vi "LINC Compile Sim Ops.vi"(1 "item formats":T2[](array[typedef])) -> (0 "sim ops":T1[](array[typedef]) {"mask" format="%02x"})   [LabVIEW 2018, in "STEPkgDriver_LINC.lvlib"]
uses:
  STEPkgDriver_LINC.lvlib
  LINC Sim Ops.ctl
  LINC Format Prototype.ctl
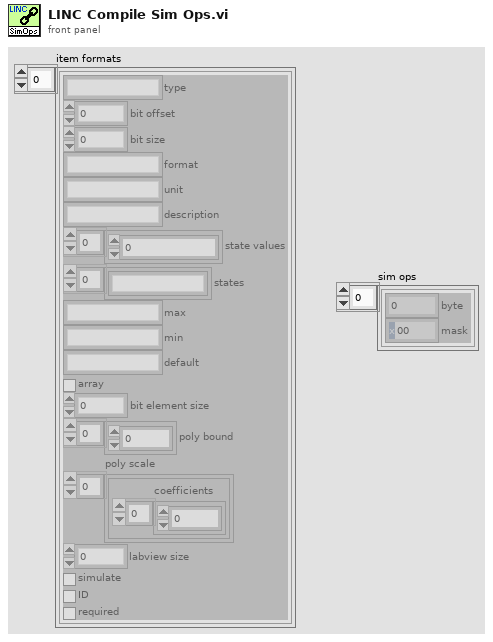
[diagram p1: front panel]
types:
  T1 = typedef "STEPkgDriver_LINC.lvlib/LINC Sim Ops.ctl" = cluster{"byte":i32, "mask":u8}
  T2 = typedef "STEPkgDriver_LINC.lvlib/LINC Format Prototype.ctl" = cluster{"type":string, "bit offset":i32, "bit size":i32, "format":string, "unit":string, "description":string, "state values":i64[], "states":string[], "max":string, "min":string, "default":string, "array":bool, "bit element size":i32, "poly bound":dbl[], "poly scale":cluster{"coefficients":dbl[]}[], "labview size":i32, "simulate":bool, "ID":bool, "required":bool}
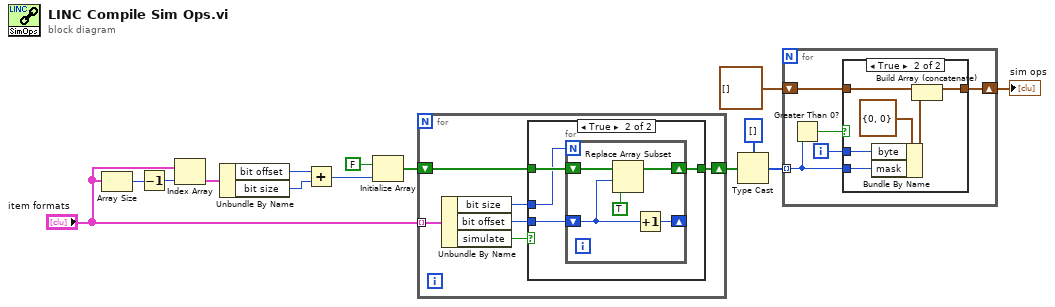
[diagram p0: block diagram]
diagram:
  n1 = Array Size(array="item formats") -> (size(s)=w14:i32)
  n2 = Decrement(x=w14) -> (x-1=w13:i32)
  n3 = Index Array(array="item formats", index=w13) -> (element=w12:T2)
  n4 = Unbundle By Name(w12) -> ("bit offset"=w11:i32, "bit size"=w10:i32)
  n5 = Add(x=w11, y=w10) -> (x+y=w9:i32)
  n6 = Initialize Array(FALSE, w9) -> (w7:bool[])
  n7 = for {
    shift-right: [w17] -> w5
    shift-left: w7 -> [w19]
    tunnel: "item formats" -> [w20] mode=indexing
    n8 = Unbundle By Name(w20) -> ("bit size"=w15:i32, "bit offset"=w16:i32, "simulate"=w18:bool)
    n9 = case shown="True" w18 {
      tunnel: w19 -> [w21 w25]
      tunnel: w15 -> [_ w24]
      tunnel: [w21 w23] -> w17
      tunnel: w16 -> [_ w22]
      frame False {
      }
      frame True {
        n10 = for {
          N: w24 -> [_]
          shift-right: [w29] -> w23
          shift-left: w25 -> [w30]
          shift-right: [w27] -> _
          shift-left: w22 -> [w28]
          n11 = Replace Array Subset(array=w30, new element=TRUE, index=w28) -> (w29:bool[])
          n12 = Increment(x=w28) -> (x+1=w27:i32)
        }
      }
    }
  }
  n13 = Type Cast(type=u8[] [], x=w5) -> (*(type *) &x=w3:u8[])
  n14 = for {
    tunnel: w3 -> [w31] mode=indexing
    shift-right: [w33] -> w1
    shift-left: T1[] [] -> [w34]
    i -> [w32]
    n15 = Greater Than 0?(x=w31) -> (x > 0?=w35:bool)
    n16 = case shown="True" w35 {
      tunnel: w34 -> [w36 w42]
      tunnel: [w36 w41] -> w33
      tunnel: w32 -> [_ w38]
      tunnel: w31 -> [_ w39]
      frame False {
      }
      frame True {
        n17 = Bundle By Name(cluster=T1 {"byte"=0, "mask"=0}, "byte"=w38, "mask"=w39) -> (w37:T1)
        n18 = Build Array (concatenate)(w42, w37) -> (w41:T1[])
      }
    }
  }
  "sim ops" <- w1
